vi "Read Applied Torque.vi"(8 "error in (no error)":errorcluster, 10 "Motor ID (0)":u8, 11 "VISA resource name":refnum<visa-resource-name>) -> (0 "error out":errorcluster, 2 "Load/torque %":sgl, 3 "VISA resource name out":refnum<visa-resource-name>)   [LabVIEW 2016, in "Dynamixel Motor.lvlib"]
doc: "Retrieves the value for the amound of torque the motor is applying."
uses:
  Dynamixel Motor.lvlib
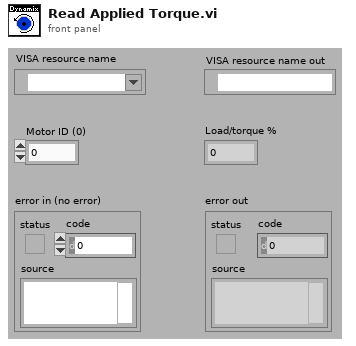
[diagram p1: front panel]
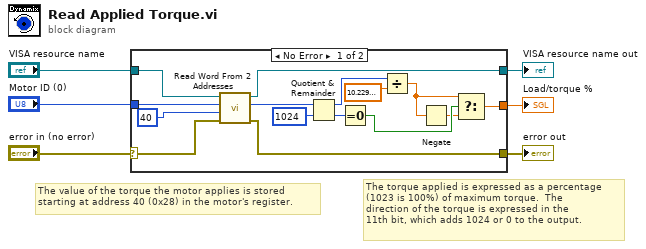
[diagram p0: block diagram]
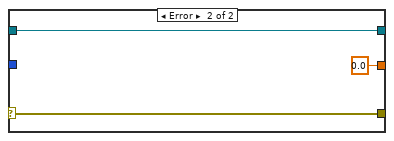
[diagram p2: hidden frame]
diagram:
  # "The torque applied is expressed as a percentage\n(1023 is 100%) of maximum torque.  The\ndirection of the torque is expressed in the \n11th bit, which adds 1024 or 0 to the output."
  # "The value of the torque the motor applies is stored\nstarting at address 40 (0x28) in the motor's register."
  n1 = case shown="No Error" "error in (no error)" {
    selector: "error in (no error)" -> [w7 w23]
    tunnel: [w17 sgl 0.0] -> w6
    tunnel: [w15 w23] -> w5
    tunnel: "VISA resource name" -> [w14 w24]
    tunnel: [w13 w24] -> w3
    tunnel: "Motor ID (0)" -> [w9 _]
    frame No Error {
      n2 = call "Read Word From 2 Addresses.vi"("Error in (no error)"=w7, "Address number (0)"=u8 40 ("Address # DEC"), "Motor ID (0)"=w9, "VISA resource name"=w14) -> ("error out"=w15:errorcluster, "Data"=w16:u16, "VISA resource name out"=w13:refnum<visa-resource-name>)  [unwired: 5 in]
      n3 = Quotient & Remainder(x=w16, y=1024) -> (x-y*floor(x/y)=w12:i32, floor(x/y)=w20:i32)
      n4 = Equal To 0?(x=w20) -> (x = 0?=w19:bool)
      n5 = Divide(x=w12, y=sgl 10.23) -> (x/y=w10:sgl)
      n6 = Negate(x=w10) -> (-x=w18:sgl)
      n7 = Select(t=w10, s=w19, f=w18) -> (s? t:f=w17:sgl)
    }
    frame Error {
    }
  }
  "VISA resource name out" <- w3
  "error out" <- w5
  "Load/torque %" <- w6
